vi "Interpret Driver Controls.vi"() -> ()   [LabVIEW 2018]
uses:
  <vilib>/Rock Robotics/WPI/DriverStation/WPI_DriverStationDerivedRobotMode.ctl
  Robot Global Data.vi
  SubSystems/Controllers/Driver Controller/Driver Controller Global.vi
  SubSystems/Drive Train/Drive Train Global.vi
  SubSystems/Lift/Lift Global.vi
  <vilib>/addons/control/pid/pid.llb/PID (DBL).vi
  SubSystems/Controllers/Manipulator Controlller/Manipulator Controller Global.vi
  SubSystems/HAB Climber/HAB Climber Global.vi
  SubSystems/Cargo Intake/Cargo Intake Global.vi
  SubSystems/Hatch Panel Intake/Hatch Panel Intake Global.vi
  <vilib>/addons/control/pid/NI_PID_pid.lvlib
panel:
  in  "Last Move Deadband":u32=500
  in  "Last Time Auto":u32=1171826
  in  "Camera Tracking":T1={"proportional gain (Kc)"=0.06, "integral time (Ti, min)"=0.0, "derivative time (Td, min)"=0.0}
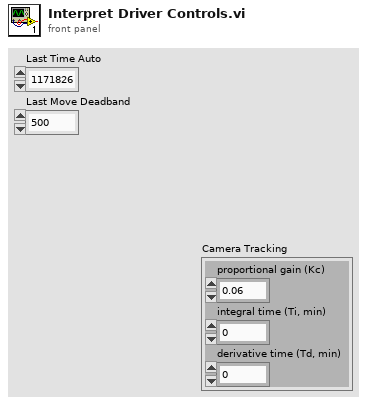
[diagram p1: front panel]
types:
  T1 = cluster{"proportional gain (Kc)":dbl, "integral time (Ti, min)":dbl, "derivative time (Td, min)":dbl}
  T2 = enum16{"Manual", "Hatch Panel Zone 1", "Hatch Panel Zone 2", "Hatch Panel Zone 3", "Cargo Zone 1", "Cargo Zone 2", "Cargo Zone 3", "Cargo Ship Zone"}
  T3 = enum16{"Hatch Panel Zone 1", "Hatch Panel Zone 2", "Hatch Panel Zone 3", "Cargo Zone 1", "Cargo Zone 2", "Cargo Zone 3", "Cargo Ship Zone"}
  T4 = cluster{"Rollover":dbl, "Yaw":dbl, "Cont Yaw":dbl}
  T5 = typedef "WPI_DriverStationDerivedRobotMode.ctl" = enum16{"Init", "Execute", "Stop"}
  T6 = cluster{"offsetAngle H":dbl, "offsetAngle V":dbl, "area":dbl, "skew":dbl, "validTarget":dbl, "latency":dbl}
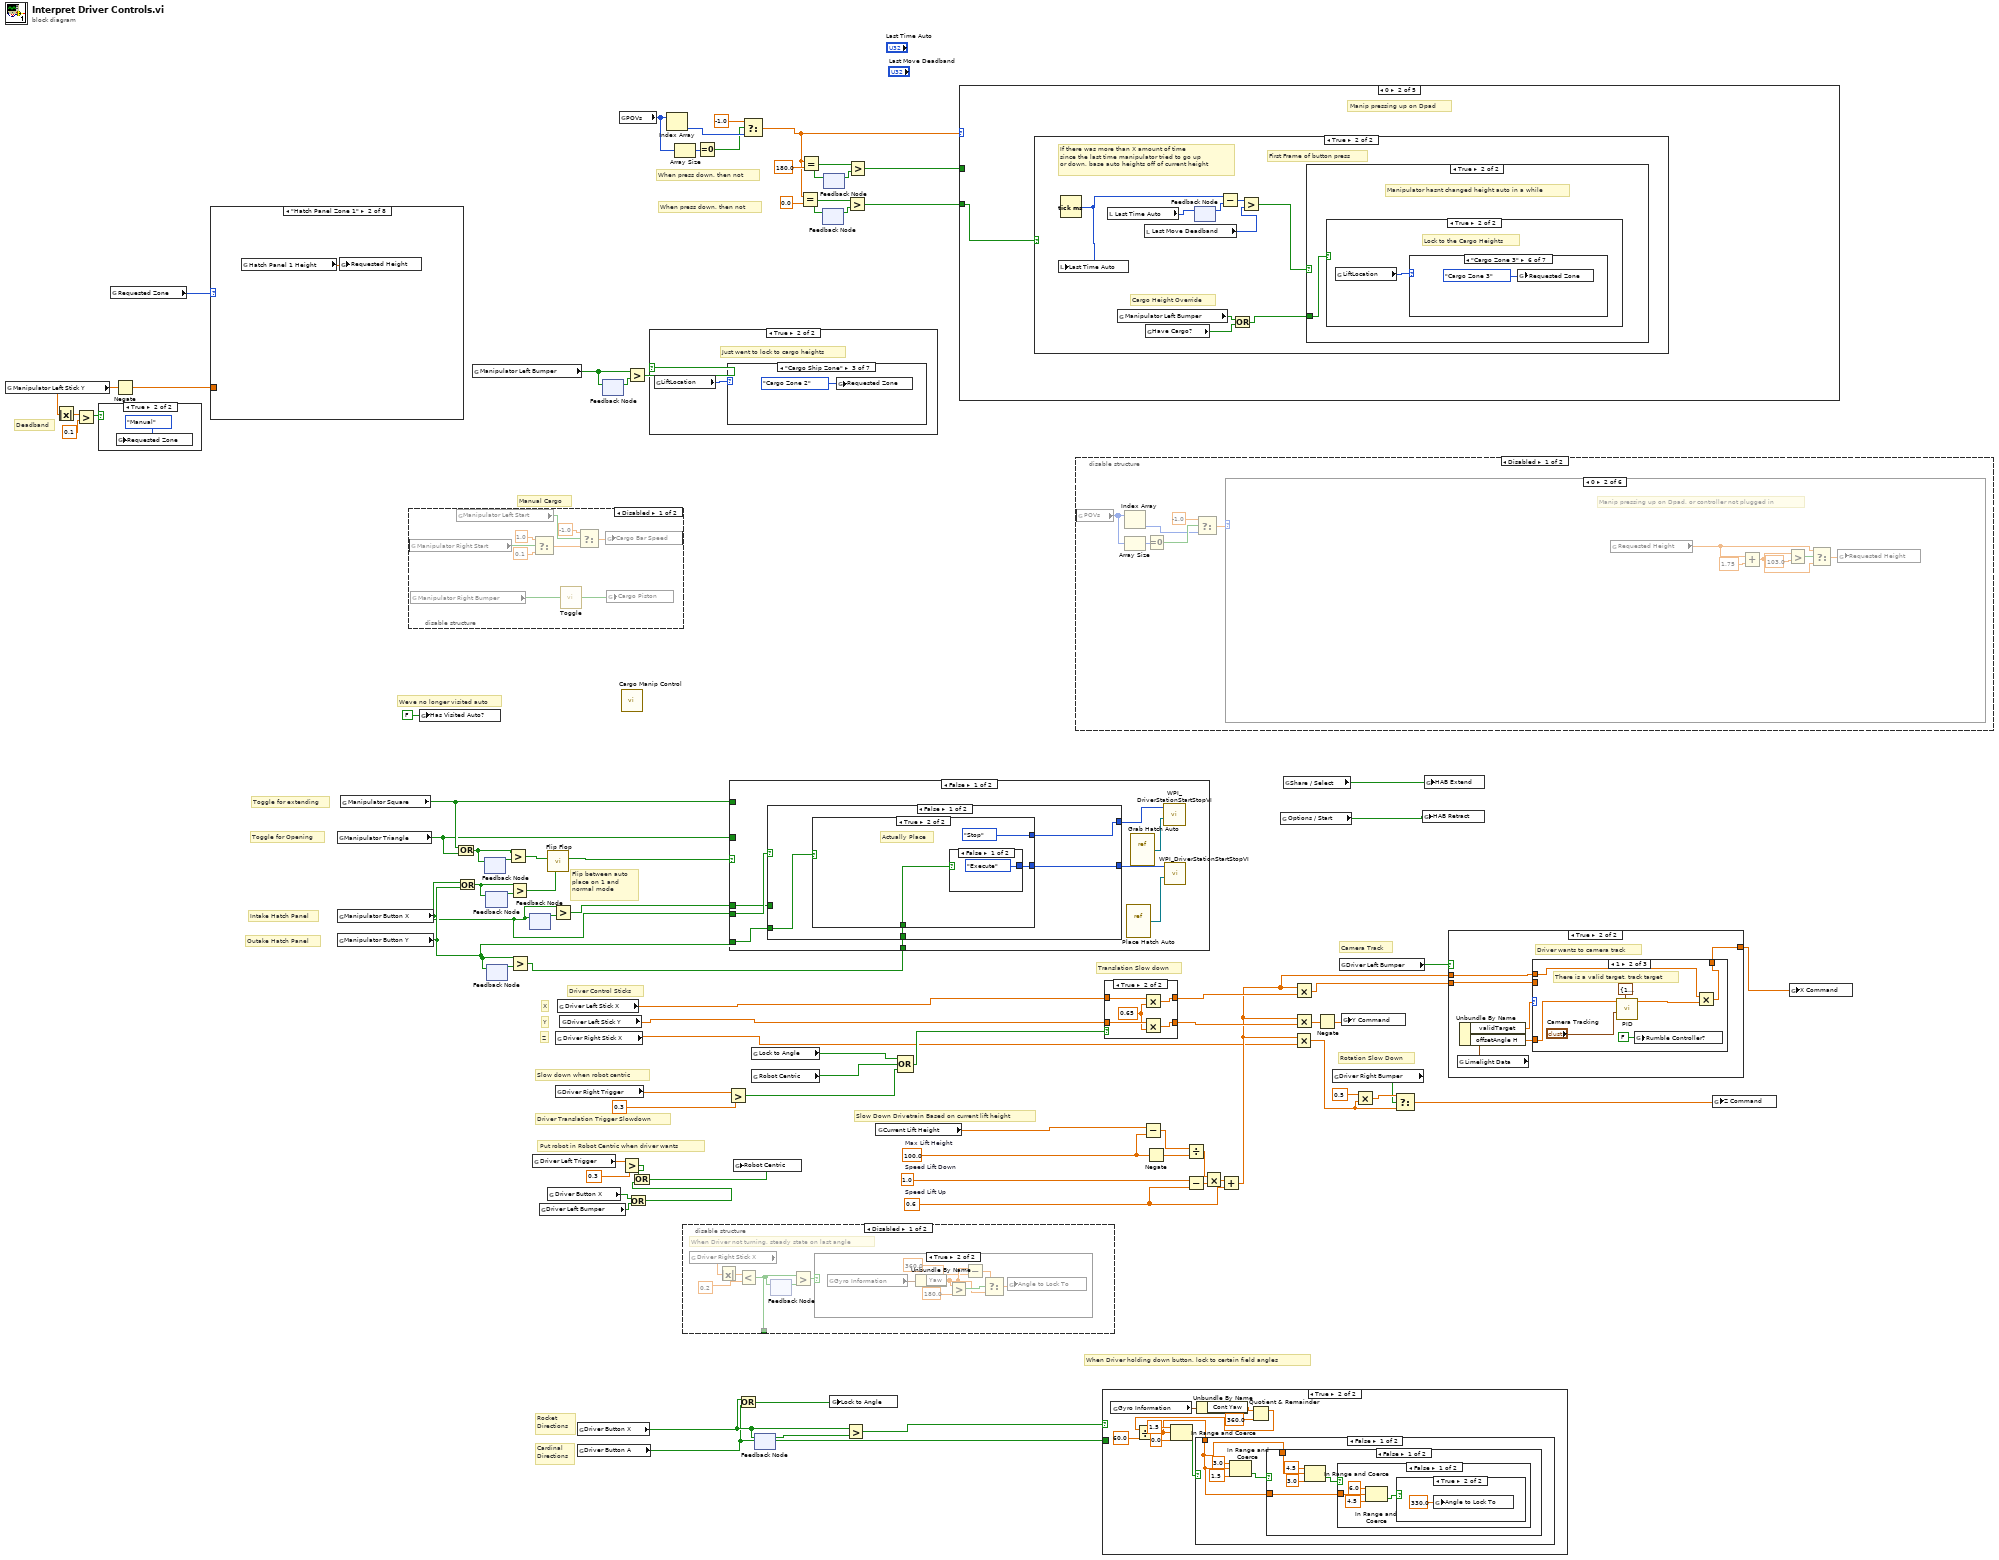
[diagram p0: block diagram]
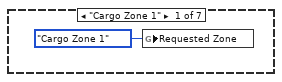
[diagram p3: hidden frame]
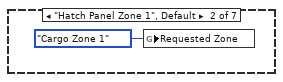
[diagram p4: hidden frame]
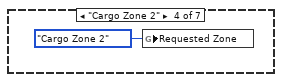
[diagram p5: hidden frame]
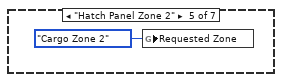
[diagram p6: hidden frame]
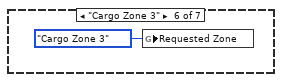
[diagram p7: hidden frame]
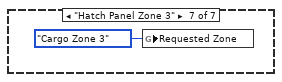
[diagram p8: hidden frame]
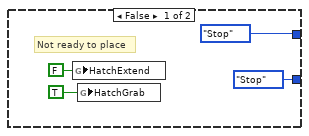
[diagram p9: hidden frame]
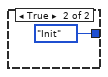
[diagram p10: hidden frame]
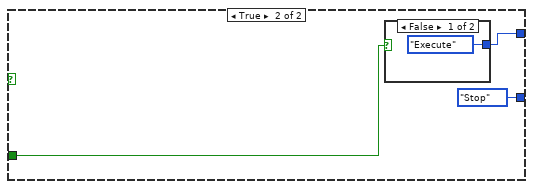
[diagram p11: hidden frame]
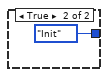
[diagram p12: hidden frame]
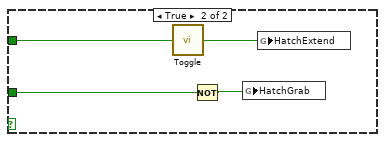
[diagram p13: hidden frame]
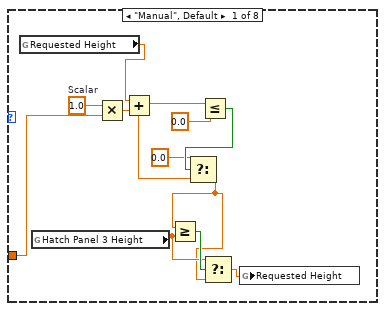
[diagram p15: hidden frame]
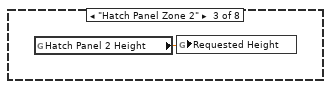
[diagram p16: hidden frame]
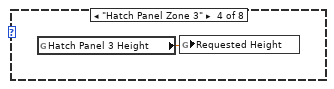
[diagram p17: hidden frame]
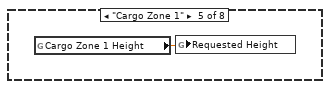
[diagram p18: hidden frame]
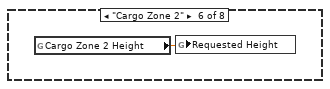
[diagram p19: hidden frame]
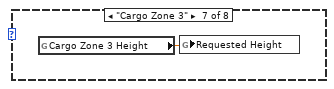
[diagram p20: hidden frame]
diagram:
  w65 = 0.6  # Speed Lift Up
  w69 = 1.0  # Speed Lift Down
  w63 = 100.0  # Max Lift Height
  # "Toggle for Opening"
  # "Toggle for extending"
  # "Outake Hatch Panel"
  # "Intake Hatch Panel"
  # "Flip between auto\nplace on 1 and \nnormal mode"
  # "When press down, then not"
  # "When press down, then not"
  # "Deadband"
  # "Manual Cargo"
  # "Weve no longer visited auto"
  # "Camera Track"
  # "Rotation Slow Down"
  # "Rocket\nDirections"
  # "Cardinal\nDirections"
  # "When Driver holding down button, lock to certain field angles"
  # "Slow Down Drivetrain Based on current lift height"
  # "Put robot in Robot Centric when driver wants"
  # "Slow down when robot centric"
  # "Driver Translation Trigger Slowdown"
  # "Translation Slow down"
  # "Z"
  # "Y"
  # "X"
  # "Driver Control Sticks"
  n1 = global read "Manipulator Controller Global.vi" "Manipulator Left Stick Y"() -> (w34:dbl)
  n2 = Absolute Value(x=w34) -> (abs(x)=w37:dbl)
  n3 = Greater?(x=w37, y=0.1) -> (0:w35:bool)
  n4 = case shown="True" w35 {
    frame False {
    }
    frame True {
      n5 = global write "Lift Global.vi" "Requested Zone"(T2."Manual" ("Requested Zone")) -> ()
    }
  }
  n6 = global read "Lift Global.vi" "Requested Zone"() -> (w38:T2)
  n7 = Negate(x=w34) -> (-x=w33:dbl)
  n8 = case shown="\"Hatch Panel Zone 1\"" w38 {
    tunnel: w33 -> [w95 _ _ _ _ _ _ _]
    frame "Manual", Default {
      w94 = 1.0  # Scalar
      n9 = global read "Lift Global.vi" "Requested Height"() -> (w97:dbl)
      n10 = global read "Lift Global.vi" "Hatch Panel 3 Height"() -> (w88:dbl)
      n11 = Multiply(x=w94, y=w95) -> (x*y=w96:dbl)
      n12 = Add(x=w97, y=w96) -> (x+y=w90:dbl)
      n13 = Less Or Equal?(x=w90, y=0.0) -> (x <= y?=w92:bool)
      n14 = Select(t=0.0, s=w92, f=w90) -> (s? t:f=w87:dbl)
      n15 = Greater Or Equal?(x=w87, y=w88) -> (x >= y?=w89:bool)
      n16 = Select(t=w88, s=w89, f=w87) -> (s? t:f=w86:dbl)
      n17 = global write "Lift Global.vi" "Requested Height"(w86) -> ()
    }
    frame "Hatch Panel Zone 1" {
      n18 = global read "Lift Global.vi" "Hatch Panel 1 Height"() -> (w98:dbl)
      n19 = global write "Lift Global.vi" "Requested Height"(w98) -> ()
    }
    frame "Hatch Panel Zone 2" {
      n20 = global read "Lift Global.vi" "Hatch Panel 2 Height"() -> (w99:dbl)
      n21 = global write "Lift Global.vi" "Requested Height"(w99) -> ()
    }
    frame "Hatch Panel Zone 3" {
      n22 = global read "Lift Global.vi" "Hatch Panel 3 Height"() -> (w100:dbl)
      n23 = global write "Lift Global.vi" "Requested Height"(w100) -> ()
    }
    frame "Cargo Zone 1" {
      n24 = global read "Lift Global.vi" "Cargo Zone 1 Height"() -> (w101:dbl)
      n25 = global write "Lift Global.vi" "Requested Height"(w101) -> ()
    }
    frame "Cargo Zone 2" {
      n26 = global read "Lift Global.vi" "Cargo Zone 2 Height"() -> (w102:dbl)
      n27 = global write "Lift Global.vi" "Requested Height"(w102) -> ()
    }
    frame "Cargo Zone 3" {
      n28 = global read "Lift Global.vi" "Cargo Zone 3 Height"() -> (w103:dbl)
      n29 = global write "Lift Global.vi" "Requested Height"(w103) -> ()
    }
    frame "Cargo Ship Zone" {
      n30 = global read "Lift Global.vi" "Cargo Ship Height"() -> (w104:dbl)
      n31 = global write "Lift Global.vi" "Requested Height"(w104) -> ()
    }
  }
  n32 = global read "Manipulator Controller Global.vi" "Manipulator Triangle"() -> (w20:bool)
  n33 = global read "Manipulator Controller Global.vi" "Manipulator Button X"() -> (w5:bool)
  n34 = global read "Manipulator Controller Global.vi" "Manipulator Button Y"() -> (w10:bool)
  n35 = global read "Manipulator Controller Global.vi" "Manipulator Square"() -> (w21:bool)
  n36 = disable-structure shown="Disabled" {
    frame Disabled {
      n37 = global read "Manipulator Controller Global.vi" "Manipulator Right Start"() -> (w110:bool)
      n38 = global read "Manipulator Controller Global.vi" "Manipulator Right Bumper"() -> (w113:bool)
      n39 = global read "Manipulator Controller Global.vi" "Manipulator Left Start"() -> (w109:bool)
      n40 = Select(t=1.0, s=w110, f=0.1) -> (s? t:f=w108:dbl)
      n41 = call "Toggle.vi"("Input"=w113) -> ("Output"=w112:bool)
      n42 = Select(t=-1.0, s=w109, f=w108) -> (s? t:f=w111:dbl)
      n43 = global write "Cargo Intake Global.vi" "Cargo Bar Speed"(w111) -> ()
      n44 = global write "Cargo Intake Global.vi" "Cargo Piston"(w112) -> ()
    }
    frame Enabled {
    }
  }
  n45 = global write "Robot Global Data.vi" "Has Visited Auto?"(FALSE ("Has Visited Auto?")) -> ()
  n46 = Or(x=w21, y=w20) -> (x .or. y?=w18:bool)
  n47 = Or(x=w5, y=w10) -> (x .or. y?=w15:bool)
  n48 = global read "Manipulator Controller Global.vi" "Manipulator Left Bumper"() -> (w2:bool)
  n49 = feedback-in #1(w18) -> ()
  n50 = feedback #1() -> (w19:bool)  [unwired: 1 in]
  n51 = feedback #2() -> (w16:bool)  [unwired: 1 in]
  n52 = feedback-in #2(w15) -> ()
  n53 = feedback #3() -> (w12:bool)  [unwired: 1 in]
  n54 = feedback-in #3(w10) -> ()
  n55 = Greater?(x=w18, y=w19) -> (0:w17:bool)
  n56 = Greater?(x=w15, y=w16) -> (0:w14:bool)
  n57 = Greater?(x=w10, y=w12) -> (0:w11:bool)
  n58 = feedback #4() -> (w6:bool)  [unwired: 1 in]
  n59 = feedback-in #4(w5) -> ()
  n60 = global read "Driver Controller Global.vi" "Driver Left Trigger"() -> (w81:dbl)
  n61 = global read "Driver Controller Global.vi" "Driver Left Bumper"() -> (w48:bool)
  n62 = call "Flip Flop.vi"("Line 2"=w14, "Line 1"=w17) -> ("Switch"=w13:bool)  [unwired: 9 in]
  n63 = global read "Driver Controller Global.vi" "Driver Button X"() -> (w49:bool)
  n64 = Greater?(x=w5, y=w6) -> (0:w4:bool)
  n65 = global read "Driver Controller Global.vi" "Driver Right Trigger"() -> (w84:dbl)
  n66 = global read "Driver Controller Global.vi" "Driver Right Stick X"() -> (w7:dbl)
  n67 = global read "Driver Controller Global.vi" "Driver Left Stick X"() -> (w9:dbl)
  n68 = global read "Driver Controller Global.vi" "Driver Left Stick Y"() -> (w8:dbl)
  n69 = global read "Driver Controller Global.vi" "Driver Button X"() -> (w61:bool)
  n70 = global read "Driver Controller Global.vi" "Driver Button A"() -> (w59:bool)
  n71 = feedback #5() -> (w3:bool)  [unwired: 1 in]
  n72 = feedback-in #5(w2) -> ()
  n73 = global read "Manipulator Controller Global.vi" "POVs"() -> (w42:i16[])
  n74 = call "Cargo Manip Control.vi"() -> ()  [unwired: 12 in]
  n75 = Greater?(x=w81, y=0.3) -> (0:w57:bool)
  n76 = Greater?(x=w2, y=w3) -> (0:w1:bool)
  n77 = Or(x=w49, y=w48) -> (x .or. y?=w50:bool)
  n78 = Or(x=w57, y=w50) -> (x .or. y?=w55:bool)
  n79 = case shown="True" w1 {
    frame False {
    }
    frame True {
      # "Just went to lock to cargo heights"
      n80 = global read "Lift Global.vi" "LiftLocation"() -> (w114:T3)
      n81 = case shown="\"Cargo Ship Zone\"" w114 {
        frame "Cargo Zone 1" {
          n82 = global write "Lift Global.vi" "Requested Zone"(T2."Cargo Zone 1" ("Requested Zone")) -> ()
        }
        frame "Hatch Panel Zone 1", Default {
          n83 = global write "Lift Global.vi" "Requested Zone"(T2."Cargo Zone 1" ("Requested Zone")) -> ()
        }
        frame "Cargo Ship Zone" {
          n84 = global write "Lift Global.vi" "Requested Zone"(T2."Cargo Zone 2" ("Requested Zone")) -> ()
        }
        frame "Cargo Zone 2" {
          n85 = global write "Lift Global.vi" "Requested Zone"(T2."Cargo Zone 2" ("Requested Zone")) -> ()
        }
        frame "Hatch Panel Zone 2" {
          n86 = global write "Lift Global.vi" "Requested Zone"(T2."Cargo Zone 2" ("Requested Zone")) -> ()
        }
        frame "Cargo Zone 3" {
          n87 = global write "Lift Global.vi" "Requested Zone"(T2."Cargo Zone 3" ("Requested Zone")) -> ()
        }
        frame "Hatch Panel Zone 3" {
          n88 = global write "Lift Global.vi" "Requested Zone"(T2."Cargo Zone 3" ("Requested Zone")) -> ()
        }
      }
    }
  }
  n89 = Index Array(array=w42) -> (element=w39:i16)  [unwired: 1 in]
  n90 = Array Size(array=w42) -> (size(s)=w41:i32)
  n91 = disable-structure shown="Disabled" {
    disable-tunnel: [w122 _] -> _
    frame Disabled {
      # "When Driver not turning, steady state on last angle"
      n92 = global read "Driver Controller Global.vi" "Driver Right Stick X"() -> (w123:dbl)
      n93 = Absolute Value(x=w123) -> (abs(x)=w127:dbl)
      n94 = Less?(x=w127, y=0.2) -> (x < y?=w122:bool)
      n95 = feedback #6() -> (w125:bool)  [unwired: 1 in]
      n96 = feedback-in #6(w122) -> ()
      n97 = Greater?(x=w122, y=w125) -> (0:w124:bool)
      n98 = case shown="True" w124 {
        frame False {
        }
        frame True {
          n99 = global read "Drive Train Global.vi" "Gyro Information"() -> (w134:T4)
          n100 = Unbundle By Name(w134) -> ("Yaw"=w131:dbl)
          n101 = Greater?(x=w131, y=180.0) -> (0:w132:bool)
          n102 = Subtract(x=w131, y=360.0) -> (x-y=w129:dbl)
          n103 = Select(t=w129, s=w132, f=w131) -> (s? t:f=w128:dbl)
          n104 = global write "Drive Train Global.vi" "Angle to Lock To"(w128) -> ()
        }
      }
    }
    frame Enabled {
    }
  }
  n105 = Equal To 0?(x=w41) -> (x = 0?=w32:bool)
  n106 = Greater?(x=w84, y=0.3) -> (0:w76:bool)
  n107 = case shown="False" w13 {
    tunnel: w20 -> [_ w162]
    tunnel: w21 -> [_ w163]
    tunnel: w5 -> [w142 _]
    tunnel: w11 -> [w139 _]
    tunnel: w10 -> [w138 _]
    tunnel: w4 -> [w135 _]
    frame False {
      n108 = case shown="False" w142 {
        tunnel: [w146 WPI_DriverStationDerivedRobotMode."Stop" ("Call Context")] -> w140
        tunnel: w139 -> [w145 _]
        tunnel: w138 -> [w144 _]
        tunnel: [w143 w157] -> w136
        tunnel: w135 -> [_ w156]
        frame False {
          n109 = case shown="True" w144 {
            tunnel: [WPI_DriverStationDerivedRobotMode."Stop" ("Call Context") w153] -> w146
            tunnel: w145 -> [_ w152]
            tunnel: [WPI_DriverStationDerivedRobotMode."Stop" ("Call Context") WPI_DriverStationDerivedRobotMode."Stop" ("Call Context")] -> w143
            frame False {
              # "Not ready to place"
              n110 = global write "Hatch Panel Intake Global.vi" "HatchExtend"(FALSE ("HatchExtend")) -> ()
              n111 = global write "Hatch Panel Intake Global.vi" "HatchGrab"(TRUE ("HatchExtend")) -> ()
            }
            frame True {
              # "Actually Place"
              n112 = case shown="False" w152 {
                tunnel: [WPI_DriverStationDerivedRobotMode."Execute" ("Call Context") WPI_DriverStationDerivedRobotMode."Init" ("Call Context")] -> w153
                frame False {
                }
                frame True {
                }
              }
            }
          }
        }
        frame True {
          n113 = case shown="False" w156 {
            tunnel: [WPI_DriverStationDerivedRobotMode."Execute" ("Call Context") WPI_DriverStationDerivedRobotMode."Init" ("Call Context")] -> w157
            frame False {
            }
            frame True {
            }
          }
        }
      }
      n114 = vi-ref "Place Hatch Auto.vi"() -> (w141:refnum<vi>)
      n115 = vi-ref "Grab Hatch Auto.vi"() -> (w137:refnum<vi>)
      n116 = call <vilib>:"WPI_DriverStationStartStopVI.vi"("VI in"=w137, "Call Context"=w136) -> ()  [unwired: 10 in]
      n117 = call <vilib>:"WPI_DriverStationStartStopVI.vi"("VI in"=w141, "Call Context"=w140) -> ()  [unwired: 10 in]
    }
    frame True {
      n118 = call "Toggle.vi"("Input"=w163) -> ("Output"=w164:bool)
      n119 = Not(x=w162) -> (.not. x?=w161:bool)
      n120 = global write "Hatch Panel Intake Global.vi" "HatchGrab"(w161) -> ()
      n121 = global write "Hatch Panel Intake Global.vi" "HatchExtend"(w164) -> ()
    }
  }
  n122 = global write "Drive Train Global.vi" "Robot Centric"(w55) -> ()
  n123 = Or(x=w61, y=w59) -> (x .or. y?=w58:bool)
  n124 = Select(t=-1.0, s=w32, f=w39) -> (s? t:f=w24:dbl)
  n125 = global read "Drive Train Global.vi" "Lock to Angle"() -> (w56:bool)
  n126 = global read "Drive Train Global.vi" "Robot Centric"() -> (w75:bool)
  n127 = feedback #7() -> (w62:bool)  [unwired: 1 in]
  n128 = feedback-in #7(w61) -> ()
  n129 = Equal?(x=w24, y=0.0) -> (x = y?=w27:bool)
  n130 = Equal?(x=w24, y=180.0) -> (x = y?=w29:bool)
  n131 = feedback #8() -> (w26:bool)  [unwired: 1 in]
  n132 = feedback-in #8(w27) -> ()
  n133 = feedback-in #9(w29) -> ()
  n134 = feedback #9() -> (w30:bool)  [unwired: 1 in]
  n135 = global write "Drive Train Global.vi" "Lock to Angle"(w58) -> ()
  n136 = Greater?(x=w61, y=w62) -> (0:w60:bool)
  n137 = Greater?(x=w27, y=w26) -> (0:w23:bool)
  n138 = Greater?(x=w29, y=w30) -> (0:w28:bool)
  n139 = global read "Lift Global.vi" "Current Lift Height"() -> (w71:dbl)
  n140 = Compound Arithmetic op=OR(w56, w75, w76) -> (w74:bool)
  n141 = case shown="0" w24 {
    tunnel: w28 -> [_ _ w209 _ _]
    tunnel: w23 -> [_ w165 _ _ _]
    frame -1, Default {
      # "Nothing on the D-Pad is pressed!"
    }
    frame 0 {
      # "Manip pressing up on Dpad"
      n142 = case shown="True" w165 {
        frame False {
          # "Still pressing button, do nothing"
        }
        frame True {
          # "Cargo Height Override"
          # "First Frame of button press"
          # "If there was more than X amount of time\nsince the last time manipulator tried to go up\nor down, base auto heights off of current height"
          n143 = Tick Count (ms)() -> (millisecond timer value=w171:u32)
          n144 = local write "Last Time Auto"(w171) -> ()
          n145 = local read "Last Time Auto"() -> (w170:u32)
          n146 = global read "Manipulator Controller Global.vi" "Manipulator Left Bumper"() -> (w168:bool)
          n147 = local read "Last Move Deadband"() -> (w172:u32)
          n148 = global read "Cargo Intake Global.vi" "Have Cargo?"() -> (w166:bool)
          n149 = feedback #10() -> (w169:u32)  [unwired: 1 in]
          n150 = feedback-in #10(w170) -> ()
          n151 = Subtract(x=w171, y=w169) -> (x-y=w174:u32)
          n152 = Or(x=w168, y=w166) -> (x .or. y?=w167:bool)
          n153 = Greater?(x=w174, y=w172) -> (0:w173:bool)
          n154 = case shown="True" w173 {
            tunnel: w167 -> [w175 w192]
            frame False {
              # "Manipulator is still changing height to go to"
              n155 = case shown="False" w175 {
                frame False {
                  # "Lock to the Hatch Heights"
                  n156 = global read "Lift Global.vi" "Requested Zone"() -> (w176:T2)
                  n157 = case shown="\"Hatch Panel Zone 3\"" w176 {
                    frame "Manual" {
                    }
                    frame "Cargo Zone 1" {
                      n158 = global write "Lift Global.vi" "Requested Zone"(T2."Hatch Panel Zone 1" ("Requested Zone")) -> ()
                    }
                    frame "Hatch Panel Zone 1", Default {
                      n159 = global write "Lift Global.vi" "Requested Zone"(T2."Hatch Panel Zone 2" ("Requested Zone")) -> ()
                    }
                    frame "Cargo Ship Zone" {
                      n160 = global write "Lift Global.vi" "Requested Zone"(T2."Hatch Panel Zone 2" ("Requested Zone")) -> ()
                    }
                    frame "Cargo Zone 2" {
                      n161 = global write "Lift Global.vi" "Requested Zone"(T2."Hatch Panel Zone 2" ("Requested Zone")) -> ()
                    }
                    frame "Hatch Panel Zone 2" {
                      n162 = global write "Lift Global.vi" "Requested Zone"(T2."Hatch Panel Zone 3" ("Requested Zone")) -> ()
                    }
                    frame "Cargo Zone 3" {
                      n163 = global write "Lift Global.vi" "Requested Zone"(T2."Hatch Panel Zone 3" ("Requested Zone")) -> ()
                    }
                    frame "Hatch Panel Zone 3" {
                      n164 = global write "Lift Global.vi" "Requested Zone"(T2."Hatch Panel Zone 3" ("Requested Zone")) -> ()
                    }
                  }
                }
                frame True {
                  # "Lock to the Cargo Heights"
                  n165 = global read "Lift Global.vi" "Requested Zone"() -> (w184:T2)
                  n166 = case shown="\"Manual\"" w184 {
                    frame "Manual" {
                    }
                    frame "Cargo Zone 1" {
                      n167 = global write "Lift Global.vi" "Requested Zone"(T2."Cargo Zone 2" ("Requested Zone")) -> ()
                    }
                    frame "Hatch Panel Zone 1", Default {
                      n168 = global write "Lift Global.vi" "Requested Zone"(T2."Cargo Zone 2" ("Requested Zone")) -> ()
                    }
                    frame "Cargo Ship Zone" {
                      n169 = global write "Lift Global.vi" "Requested Zone"(T2."Cargo Zone 2" ("Requested Zone")) -> ()
                    }
                    frame "Cargo Zone 2" {
                      n170 = global write "Lift Global.vi" "Requested Zone"(T2."Cargo Zone 3" ("Requested Zone")) -> ()
                    }
                    frame "Hatch Panel Zone 2" {
                      n171 = global write "Lift Global.vi" "Requested Zone"(T2."Cargo Zone 3" ("Requested Zone")) -> ()
                    }
                    frame "Cargo Zone 3" {
                      n172 = global write "Lift Global.vi" "Requested Zone"(T2."Cargo Zone 3" ("Requested Zone")) -> ()
                    }
                    frame "Hatch Panel Zone 3" {
                      n173 = global write "Lift Global.vi" "Requested Zone"(T2."Cargo Zone 3" ("Requested Zone")) -> ()
                    }
                  }
                }
              }
            }
            frame True {
              # "Manipulator hasnt changed height auto in a while"
              n174 = case shown="True" w192 {
                frame False {
                  # "Lock to the Hatch Heights"
                  n175 = global read "Lift Global.vi" "LiftLocation"() -> (w193:T3)
                  n176 = case shown="\"Cargo Zone 1\"" w193 {
                    frame "Cargo Zone 1" {
                      n177 = global write "Lift Global.vi" "Requested Zone"(T2."Hatch Panel Zone 1" ("Requested Zone")) -> ()
                    }
                    frame "Hatch Panel Zone 1", Default {
                      n178 = global write "Lift Global.vi" "Requested Zone"(T2."Hatch Panel Zone 2" ("Requested Zone")) -> ()
                    }
                    frame "Cargo Ship Zone" {
                      n179 = global write "Lift Global.vi" "Requested Zone"(T2."Hatch Panel Zone 2" ("Requested Zone")) -> ()
                    }
                    frame "Cargo Zone 2" {
                      n180 = global write "Lift Global.vi" "Requested Zone"(T2."Hatch Panel Zone 2" ("Requested Zone")) -> ()
                    }
                    frame "Hatch Panel Zone 2" {
                      n181 = global write "Lift Global.vi" "Requested Zone"(T2."Hatch Panel Zone 3" ("Requested Zone")) -> ()
                    }
                    frame "Cargo Zone 3" {
                      n182 = global write "Lift Global.vi" "Requested Zone"(T2."Hatch Panel Zone 3" ("Requested Zone")) -> ()
                    }
                    frame "Hatch Panel Zone 3" {
                      n183 = global write "Lift Global.vi" "Requested Zone"(T2."Hatch Panel Zone 3" ("Requested Zone")) -> ()
                    }
                  }
                }
                frame True {
                  # "Lock to the Cargo Heights"
                  n184 = global read "Lift Global.vi" "LiftLocation"() -> (w201:T3)
                  n185 = case shown="\"Cargo Zone 3\"" w201 {
                    frame "Cargo Zone 1" {
                      n186 = global write "Lift Global.vi" "Requested Zone"(T2."Cargo Zone 2" ("Requested Zone")) -> ()
                    }
                    frame "Hatch Panel Zone 1", Default {
                      n187 = global write "Lift Global.vi" "Requested Zone"(T2."Cargo Zone 2" ("Requested Zone")) -> ()
                    }
                    frame "Cargo Ship Zone" {
                      n188 = global write "Lift Global.vi" "Requested Zone"(T2."Cargo Zone 2" ("Requested Zone")) -> ()
                    }
                    frame "Cargo Zone 2" {
                      n189 = global write "Lift Global.vi" "Requested Zone"(T2."Cargo Zone 3" ("Requested Zone")) -> ()
                    }
                    frame "Hatch Panel Zone 2" {
                      n190 = global write "Lift Global.vi" "Requested Zone"(T2."Cargo Zone 3" ("Requested Zone")) -> ()
                    }
                    frame "Cargo Zone 3" {
                      n191 = global write "Lift Global.vi" "Requested Zone"(T2."Cargo Zone 3" ("Requested Zone")) -> ()
                    }
                    frame "Hatch Panel Zone 3" {
                      n192 = global write "Lift Global.vi" "Requested Zone"(T2."Cargo Zone 3" ("Requested Zone")) -> ()
                    }
                  }
                }
              }
            }
          }
        }
      }
    }
    frame 180 {
      # "Manip pressing down on Dpad"
      n193 = case shown="True" w209 {
        frame False {
          # "Still pressing button, do nothing"
        }
        frame True {
          # "Cargo Height Override"
          # "First frame of button press"
          # "If there was more than X amount of time\nsince the last time manipulator tried to go up\nor down, base auto heights off of current height"
          n194 = Tick Count (ms)() -> (millisecond timer value=w217:u32)
          n195 = local write "Last Time Auto"(w217) -> ()
          n196 = local read "Last Time Auto"() -> (w215:u32)
          n197 = global read "Manipulator Controller Global.vi" "Manipulator Left Bumper"() -> (w212:bool)
          n198 = local read "Last Move Deadband"() -> (w216:u32)
          n199 = global read "Cargo Intake Global.vi" "Have Cargo?"() -> (w211:bool)
          n200 = feedback #11() -> (w214:u32)  [unwired: 1 in]
          n201 = feedback-in #11(w215) -> ()
          n202 = Subtract(x=w217, y=w214) -> (x-y=w218:u32)
          n203 = Greater?(x=w218, y=w216) -> (0:w213:bool)
          n204 = Or(x=w212, y=w211) -> (x .or. y?=w210:bool)
          n205 = case shown="False" w213 {
            tunnel: w210 -> [w219 w236]
            frame False {
              # "Manipulator is still changing height to go to"
              n206 = case shown="False" w219 {
                frame False {
                  # "Lock to the Hatch Heights"
                  n207 = global read "Lift Global.vi" "Requested Zone"() -> (w220:T2)
                  n208 = case shown="\"Hatch Panel Zone 3\"" w220 {
                    frame "Manual" {
                    }
                    frame "Cargo Zone 1" {
                      n209 = global write "Lift Global.vi" "Requested Zone"(T2."Hatch Panel Zone 1" ("Requested Zone")) -> ()
                    }
                    frame "Hatch Panel Zone 1", Default {
                      n210 = global write "Lift Global.vi" "Requested Zone"(T2."Hatch Panel Zone 1" ("Requested Zone")) -> ()
                    }
                    frame "Cargo Ship Zone" {
                      n211 = global write "Lift Global.vi" "Requested Zone"(T2."Hatch Panel Zone 1" ("Requested Zone")) -> ()
                    }
                    frame "Cargo Zone 2" {
                      n212 = global write "Lift Global.vi" "Requested Zone"(T2."Hatch Panel Zone 1" ("Requested Zone")) -> ()
                    }
                    frame "Hatch Panel Zone 2" {
                      n213 = global write "Lift Global.vi" "Requested Zone"(T2."Hatch Panel Zone 1" ("Requested Zone")) -> ()
                    }
                    frame "Cargo Zone 3" {
                      n214 = global write "Lift Global.vi" "Requested Zone"(T2."Hatch Panel Zone 2" ("Requested Zone")) -> ()
                    }
                    frame "Hatch Panel Zone 3" {
                      n215 = global write "Lift Global.vi" "Requested Zone"(T2."Hatch Panel Zone 2" ("Requested Zone")) -> ()
                    }
                  }
                }
                frame True {
                  # "Lock to the Cargo Heights"
                  n216 = global read "Lift Global.vi" "Requested Zone"() -> (w228:T2)
                  n217 = case shown="\"Manual\"" w228 {
                    frame "Manual" {
                    }
                    frame "Cargo Zone 1" {
                      n218 = global write "Lift Global.vi" "Requested Zone"(T2."Cargo Zone 1" ("Requested Zone")) -> ()
                    }
                    frame "Hatch Panel Zone 1", Default {
                      n219 = global write "Lift Global.vi" "Requested Zone"(T2."Cargo Zone 1" ("Requested Zone")) -> ()
                    }
                    frame "Cargo Ship Zone" {
                      n220 = global write "Lift Global.vi" "Requested Zone"(T2."Cargo Zone 1" ("Requested Zone")) -> ()
                    }
                    frame "Cargo Zone 2" {
                      n221 = global write "Lift Global.vi" "Requested Zone"(T2."Cargo Zone 1" ("Requested Zone")) -> ()
                    }
                    frame "Hatch Panel Zone 2" {
                      n222 = global write "Lift Global.vi" "Requested Zone"(T2."Cargo Zone 2" ("Requested Zone")) -> ()
                    }
                    frame "Cargo Zone 3" {
                      n223 = global write "Lift Global.vi" "Requested Zone"(T2."Cargo Zone 2" ("Requested Zone")) -> ()
                    }
                    frame "Hatch Panel Zone 3" {
                      n224 = global write "Lift Global.vi" "Requested Zone"(T2."Cargo Zone 3" ("Requested Zone")) -> ()
                    }
                  }
                }
              }
            }
            frame True {
              # "Manipulator hasnt changed height auto in a while"
              n225 = case shown="False" w236 {
                frame False {
                  # "Lock to the Hatch Heights"
                  n226 = global read "Lift Global.vi" "LiftLocation"() -> (w237:T3)
                  n227 = case shown="\"Hatch Panel Zone 3\"" w237 {
                    frame "Cargo Zone 1" {
                      n228 = global write "Lift Global.vi" "Requested Zone"(T2."Hatch Panel Zone 1" ("Requested Zone")) -> ()
                    }
                    frame "Hatch Panel Zone 1", Default {
                      n229 = global write "Lift Global.vi" "Requested Zone"(T2."Hatch Panel Zone 1" ("Requested Zone")) -> ()
                    }
                    frame "Cargo Ship Zone" {
                      n230 = global write "Lift Global.vi" "Requested Zone"(T2."Hatch Panel Zone 1" ("Requested Zone")) -> ()
                    }
                    frame "Cargo Zone 2" {
                      n231 = global write "Lift Global.vi" "Requested Zone"(T2."Hatch Panel Zone 1" ("Requested Zone")) -> ()
                    }
                    frame "Hatch Panel Zone 2" {
                      n232 = global write "Lift Global.vi" "Requested Zone"(T2."Hatch Panel Zone 1" ("Requested Zone")) -> ()
                    }
                    frame "Cargo Zone 3" {
                      n233 = global write "Lift Global.vi" "Requested Zone"(T2."Hatch Panel Zone 2" ("Requested Zone")) -> ()
                    }
                    frame "Hatch Panel Zone 3" {
                      n234 = global write "Lift Global.vi" "Requested Zone"(T2."Hatch Panel Zone 2" ("Requested Zone")) -> ()
                    }
                  }
                }
                frame True {
                  # "Lock to the Cargo Heights"
                  n235 = global read "Lift Global.vi" "LiftLocation"() -> (w245:T3)
                  n236 = case shown="\"Hatch Panel Zone 3\"" w245 {
                    frame "Cargo Zone 1" {
                      n237 = global write "Lift Global.vi" "Requested Zone"(T2."Cargo Zone 1" ("Requested Zone")) -> ()
                    }
                    frame "Hatch Panel Zone 1", Default {
                      n238 = global write "Lift Global.vi" "Requested Zone"(T2."Cargo Zone 1" ("Requested Zone")) -> ()
                    }
                    frame "Cargo Ship Zone" {
                      n239 = global write "Lift Global.vi" "Requested Zone"(T2."Cargo Zone 1" ("Requested Zone")) -> ()
                    }
                    frame "Cargo Zone 2" {
                      n240 = global write "Lift Global.vi" "Requested Zone"(T2."Cargo Zone 1" ("Requested Zone")) -> ()
                    }
                    frame "Hatch Panel Zone 2" {
                      n241 = global write "Lift Global.vi" "Requested Zone"(T2."Cargo Zone 2" ("Requested Zone")) -> ()
                    }
                    frame "Cargo Zone 3" {
                      n242 = global write "Lift Global.vi" "Requested Zone"(T2."Cargo Zone 2" ("Requested Zone")) -> ()
                    }
                    frame "Hatch Panel Zone 3" {
                      n243 = global write "Lift Global.vi" "Requested Zone"(T2."Cargo Zone 3" ("Requested Zone")) -> ()
                    }
                  }
                }
              }
            }
          }
        }
      }
    }
    frame 90 {
      # "Go to Cargo in Cargo Ship Height"
      # "Right on D-Pad"
      n244 = global write "Lift Global.vi" "Requested Zone"(T2."Cargo Ship Zone" ("Requested Zone")) -> ()
    }
    frame 270 {
      # "Go to Hatch Level 1 Height"
      # "Left on D-Pad"
      n245 = global write "Lift Global.vi" "Requested Zone"(T2."Hatch Panel Zone 1" ("Requested Zone")) -> ()
    }
  }
  n246 = disable-structure shown="Disabled" {
    frame Disabled {
      n247 = global read "Manipulator Controller Global.vi" "POVs"() -> (w260:i16[])
      n248 = Index Array(array=w260) -> (element=w255:i16)  [unwired: 1 in]
      n249 = Array Size(array=w260) -> (size(s)=w259:i32)
      n250 = Equal To 0?(x=w259) -> (x = 0?=w257:bool)
      n251 = Select(t=-1.0, s=w257, f=w255) -> (s? t:f=w258:dbl)
      n252 = case shown="0" w258 {
        frame -1 {
          # "If the value changed (manip pressed button)\nchange set lift height to match"
          # "When button goes from\nnot pressed to pressed"
          n253 = global read "Manipulator Controller Global.vi" "Manipulator Square"() -> (w266:bool)
          n254 = feedback #12() -> (w267:bool)  [unwired: 1 in]
          n255 = feedback-in #12(w266) -> ()
          n256 = Greater?(x=w266, y=w267) -> (0:w263:bool)
          n257 = feedback #13() -> (w261:dbl)  [unwired: 1 in]
          n258 = feedback #14() -> (w265:dbl)  [unwired: 1 in]
          n259 = case shown="False" w263 {
            tunnel: [w277 w292] -> w262
            tunnel: w265 -> [w278 w291]
            frame False {
              # "When button goes from\nnot pressed to pressed"
              n260 = global read "Manipulator Controller Global.vi" "Manipulator Triangle"() -> (w280:bool)
              n261 = feedback #15() -> (w279:bool)  [unwired: 1 in]
              n262 = feedback-in #15(w280) -> ()
              n263 = Greater?(x=w280, y=w279) -> (0:w276:bool)
              n264 = case shown="True" w276 {
                tunnel: w278 -> [w281 w283]
                tunnel: [w281 w285] -> w277
                frame False {
                }
                frame True {
                  # "If counter smaller than 5\nadd 1"
                  n265 = Less?(x=w283, y=5.0) -> (x < y?=w282:bool)
                  n266 = case shown="True" w282 {
                    tunnel: [w286 w288] -> w285
                    tunnel: w283 -> [w286 w287]
                    frame False {
                    }
                    frame True {
                      n267 = Increment(x=w287) -> (x+1=w288:dbl)
                    }
                  }
                }
              }
            }
            frame True {
              # "If counter bigger than 0\nsubtract 1"
              n268 = Greater?(x=w291, y=0.0) -> (0:w290:bool)
              n269 = case shown="False" w290 {
                tunnel: [0.0 ("y") w295] -> w292
                tunnel: w291 -> [_ w294]
                frame False {
                }
                frame True {
                  n270 = Decrement(x=w294) -> (x-1=w295:dbl)
                }
              }
            }
          }
          n271 = feedback-in #13(w262) -> ()
          n272 = Not Equal?(x=w262, y=w261) -> (x != y?=w264:bool)
          n273 = case shown="True" w264 {
            tunnel: w262 -> [_ w268]
            frame False {
              # "Manipulator didnt request change"
            }
            frame True {
              # "Set height request to new value"
              n274 = case shown="0, Default" w268 {
                tunnel: [w270 w271 w272 w273 w274 w275] -> w269
                frame 0, Default {
                  n275 = global read "Lift Global.vi" "Cargo Zone 1 Height"() -> (w270:dbl)
                }
                frame 1 {
                  n276 = global read "Lift Global.vi" "Hatch Panel 1 Height"() -> (w271:dbl)
                }
                frame 2 {
                  n277 = global read "Lift Global.vi" "Cargo Zone 2 Height"() -> (w272:dbl)
                }
                frame 3 {
                  n278 = global read "Lift Global.vi" "Hatch Panel 2 Height"() -> (w273:dbl)
                }
                frame 4 {
                  n279 = global read "Lift Global.vi" "Cargo Zone 3 Height"() -> (w274:dbl)
                }
                frame 5 {
                  n280 = global read "Lift Global.vi" "Hatch Panel 3 Height"() -> (w275:dbl)
                }
              }
              n281 = global write "Lift Global.vi" "Requested Height"(w269) -> ()
            }
          }
          n282 = global write "Lift Global.vi" "Lift Auto Position"(w262) -> ()
          n283 = feedback-in #14(w262) -> ()
        }
        frame 0 {
          # "Manip pressing up on Dpad, or controller not plugged in"
          n284 = global read "Lift Global.vi" "Requested Height"() -> (w297:dbl)
          n285 = Add(x=w297, y=1.75) -> (x+y=w296:dbl)
          n286 = Greater?(x=w296, y=103.0) -> (0:w298:bool)
          n287 = Select(t=w297, s=w298, f=w296) -> (s? t:f=w299:dbl)
          n288 = global write "Lift Global.vi" "Requested Height"(w299) -> ()
        }
        frame 180 {
          # "Manip pressing down on Dpad"
          n289 = global read "Lift Global.vi" "Requested Height"() -> (w302:dbl)
          n290 = Add(x=w302, y=-1.0) -> (x+y=w304:dbl)
          n291 = Less?(x=w304, y=0.0) -> (x < y?=w305:bool)
          n292 = Select(t=w302, s=w305, f=w304) -> (s? t:f=w303:dbl)
          n293 = global write "Lift Global.vi" "Requested Height"(w303) -> ()
        }
        frame 90 {
          # "Go to Cargo in Cargo Ship Height"
          # "Right on D-Pad"
          n294 = global read "Lift Global.vi" "Cargo Ship Height"() -> (w308:dbl)
          n295 = global write "Lift Global.vi" "Requested Height"(w308) -> ()
        }
        frame 270 {
          # "Go to Hatch Level 1 Height"
          # "Left on D-Pad"
          n296 = global read "Lift Global.vi" "Hatch Panel 1 Height"() -> (w309:dbl)
          n297 = global write "Lift Global.vi" "Requested Height"(w309) -> ()
        }
        frame -100, Default {
        }
      }
    }
    frame Enabled {
    }
  }
  n298 = case shown="True" w60 {
    tunnel: w59 -> [w311 _]
    frame False {
      n299 = feedback #16() -> (w312:bool)  [unwired: 1 in]
      n300 = feedback-in #16(w311) -> ()
      n301 = Greater?(x=w311, y=w312) -> (0:w310:bool)
      n302 = case shown="True" w310 {
        frame False {
        }
        frame True {
          n303 = global read "Drive Train Global.vi" "Gyro Information"() -> (w319:T4)
          n304 = Unbundle By Name(w319) -> ("Yaw"=w316:dbl)
          n305 = Add(x=w316, y=180.0) -> (x+y=w315:dbl)
          n306 = Divide(x=w315, y=90.0) -> (x/y=w317:dbl)
          n307 = Round To Nearest(number=w317) -> (nearest integer value=w313:dbl)
          n308 = case shown="1" w313 {
            frame 0, Default {
              n309 = global write "Drive Train Global.vi" "Angle to Lock To"(180.0 ("Angle to Lock To")) -> ()
            }
            frame 1 {
              n310 = global write "Drive Train Global.vi" "Angle to Lock To"(270.0 ("Angle to Lock To")) -> ()
            }
            frame 2 {
              n311 = global write "Drive Train Global.vi" "Angle to Lock To"(0.0 ("Angle to Lock To")) -> ()
            }
            frame 3 {
              n312 = global write "Drive Train Global.vi" "Angle to Lock To"(90.0 ("Angle to Lock To")) -> ()
            }
            frame 4 {
              n313 = global write "Drive Train Global.vi" "Angle to Lock To"(180.0 ("Angle to Lock To")) -> ()
            }
          }
        }
      }
    }
    frame True {
      n314 = global read "Drive Train Global.vi" "Gyro Information"() -> (w333:T4)
      n315 = Unbundle By Name(w333) -> ("Cont Yaw"=w331:dbl)
      n316 = Quotient & Remainder(x=w331, y=360.0) -> (x-y*floor(x/y)=w329:dbl)  [unwired: 1 out]
      n317 = Divide(x=w329, y=60.0) -> (x/y=w325:dbl)
      n318 = In Range and Coerce(upper limit=1.5, x=w325, lower limit=0.0) -> (In Range?=w326:bool)  [unwired: 1 out]
      n319 = case shown="False" w326 {
        tunnel: w325 -> [w334 _]
        frame False {
          n320 = In Range and Coerce(upper limit=3.0, x=w334, lower limit=1.5) -> (In Range?=w335:bool)  [unwired: 1 out]
          n321 = case shown="False" w335 {
            tunnel: w334 -> [w340 _]
            tunnel: w334 -> [w338 _]
            frame False {
              n322 = In Range and Coerce(upper limit=4.5, x=w340, lower limit=3.0) -> (In Range?=w339:bool)  [unwired: 1 out]
              n323 = case shown="False" w339 {
                tunnel: w338 -> [w344 _]
                frame False {
                  n324 = In Range and Coerce(upper limit=6.0, x=w344, lower limit=4.5) -> (In Range?=w343:bool)  [unwired: 1 out]
                  n325 = case shown="True" w343 {
                    frame False {
                    }
                    frame True {
                      n326 = global write "Drive Train Global.vi" "Angle to Lock To"(330.0 ("Angle to Lock To")) -> ()
                    }
                  }
                }
                frame True {
                  n327 = global write "Drive Train Global.vi" "Angle to Lock To"(210.0 ("Angle to Lock To")) -> ()
                }
              }
            }
            frame True {
              n328 = global write "Drive Train Global.vi" "Angle to Lock To"(150.0 ("Angle to Lock To")) -> ()
            }
          }
        }
        frame True {
          n329 = global write "Drive Train Global.vi" "Angle to Lock To"(30.0 ("Angle to Lock To")) -> ()
        }
      }
    }
  }
  n330 = case shown="True" w74 {
    tunnel: w8 -> [w352 w357]
    tunnel: [w352 w356] -> w73
    tunnel: [w351 w355] -> w72
    tunnel: w9 -> [w351 w354]
    frame False {
    }
    frame True {
      w353 = 0.65 ("Y Slower")
      n331 = Multiply(x=w354, y=w353) -> (x*y=w355:dbl)
      n332 = Multiply(x=w357, y=w353) -> (x*y=w356:dbl)
    }
  }
  n333 = Subtract(x=w71, y=w63) -> (x-y=w70:dbl)
  n334 = Negate(x=w63) -> (-x=w64:dbl)
  n335 = Divide(x=w70, y=w64) -> (x/y=w68:dbl)
  n336 = Subtract(x=w69, y=w65) -> (x-y=w67:dbl)
  n337 = Multiply(x=w68, y=w67) -> (x*y=w66:dbl)
  n338 = Add(x=w66, y=w65) -> (x+y=w22:dbl)
  n339 = global read "Manipulator Controller Global.vi" "Options / Start"() -> (w46:bool)
  n340 = global read "Manipulator Controller Global.vi" "Share / Select"() -> (w47:bool)
  n341 = Multiply(x=w22, y=w7) -> (x*y=w80:dbl)
  n342 = Multiply(x=w22, y=w72) -> (x*y=w52:dbl)
  n343 = Multiply(x=w22, y=w73) -> (x*y=w45:dbl)
  n344 = Negate(x=w45) -> (-x=w44:dbl)
  n345 = global read "Driver Controller Global.vi" "Driver Right Bumper"() -> (w77:bool)
  n346 = global read "Driver Controller Global.vi" "Driver Left Bumper"() -> (w54:bool)
  n347 = global write "Drive Train Global.vi" "Y Command"(w44) -> ()
  n348 = Multiply(x=0.5, y=w80) -> (x*y=w79:dbl)
  n349 = Select(t=w79, s=w77, f=w80) -> (s? t:f=w53:dbl)
  n350 = global write "HAB Climber Global.vi" "HAB Retract"(w46) -> ()
  n351 = global write "HAB Climber Global.vi" "HAB Extend"(w47) -> ()
  n352 = case shown="True" w54 {
    tunnel: w52 -> [w359 w363]
    tunnel: [w359 w361] -> w51
    tunnel: w22 -> [_ w360]
    frame False {
      # "Driver not attepting to camera track, be normal"
      n353 = global write "Driver Controller Global.vi" "Rumble Controller?"(FALSE ("Rumble Controller?")) -> ()
    }
    frame True {
      # "Driver wants to camera track"
      n354 = global read "Robot Global Data.vi" "Limelight Data"() -> (w365:T6)
      n355 = Unbundle By Name(w365) -> ("validTarget"=w364:dbl, "offsetAngle H"=w362:dbl)
      n356 = case shown="1" w364 {
        tunnel: w363 -> [w366 _ _]
        tunnel: w362 -> [_ w371 w376]
        tunnel: [w366 w370 w377] -> w361
        tunnel: w360 -> [_ w368 _]
        frame 0, Default {
          # "No Valid Target, keep using driver controls\nand rumble controller so knows not tracking"
          n357 = global write "Driver Controller Global.vi" "Rumble Controller?"(TRUE ("Rumble Controller?")) -> ()
        }
        frame 1 {
          # "There is a valid target, track target"
          n358 = call-poly <vilib>:"PID.vi"("output range"=cluster{"output high":dbl, "output low":dbl} {"output high"=1.0, "output low"=-1.0}, "PID gains"="Camera Tracking", "setpoint"=w371) -> ("output"=w369:dbl)  [unwired: 7 in, 1 out]
          n359 = global write "Driver Controller Global.vi" "Rumble Controller?"(FALSE ("Rumble Controller?")) -> ()
          n360 = Multiply(x=w368, y=w369) -> (x*y=w370:dbl)
        }
        frame 2 {
          n361 = Multiply(x=0.1, y=w376) -> (x*y=w377:dbl)
        }
      }
    }
  }
  n362 = global write "Drive Train Global.vi" "Z Command"(w53) -> ()
  n363 = global write "Drive Train Global.vi" "X Command"(w51) -> ()
